vi "Sand Fall Till the Void.vi"(3 "Possible Movements":cdb[](array[numeric]), 4 "Sand Source Coordinates":cdb, 5 "Rock Grid":set{cdb}(c389)) -> (0 "Bounds":T1, 1 "Sand Fall steps":T2(array[cluster]), 2 "Sand Grid":set{cdb}(c389))   [LabVIEW 2020, in "AoC 2022.lvlib"]
uses:
  AoC 2022.lvlib
panel:
  out "size":i32
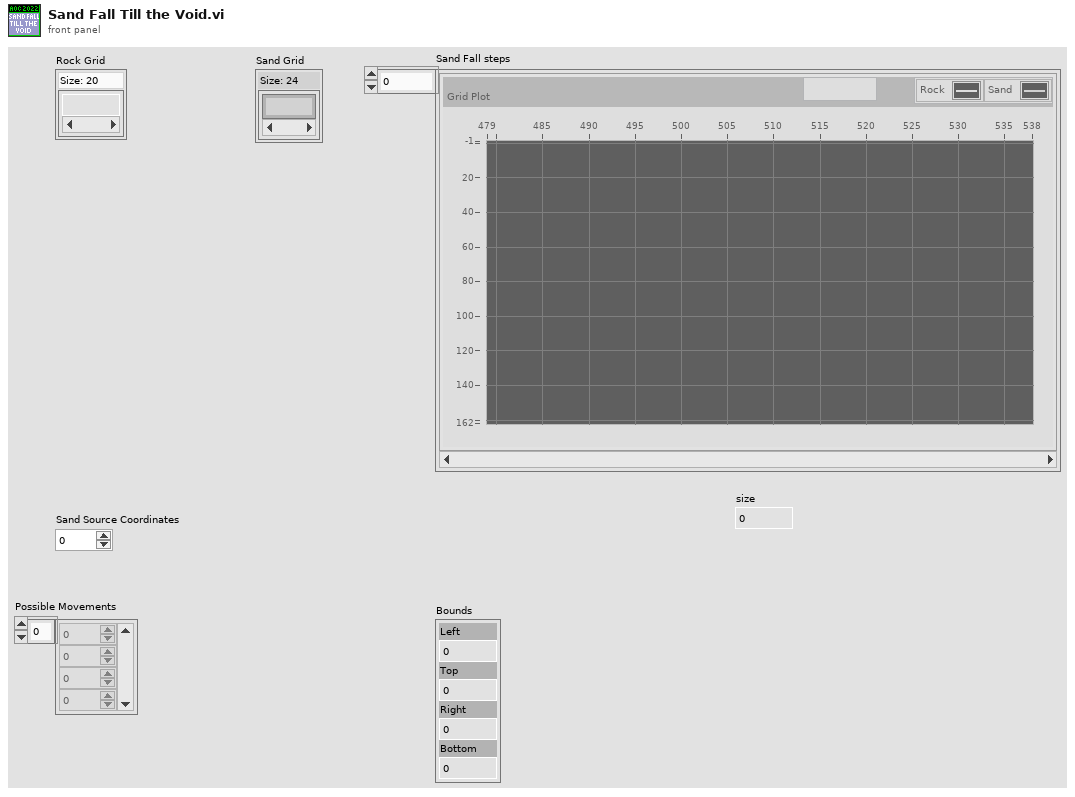
[diagram p1: front panel]
types:
  T1 = cluster{"Left":i16, "Top":i16, "Right":i16, "Bottom":i16}
  T2 = cluster{"Grid Plot":cluster{cluster{i32, i32}[]}[]}[]
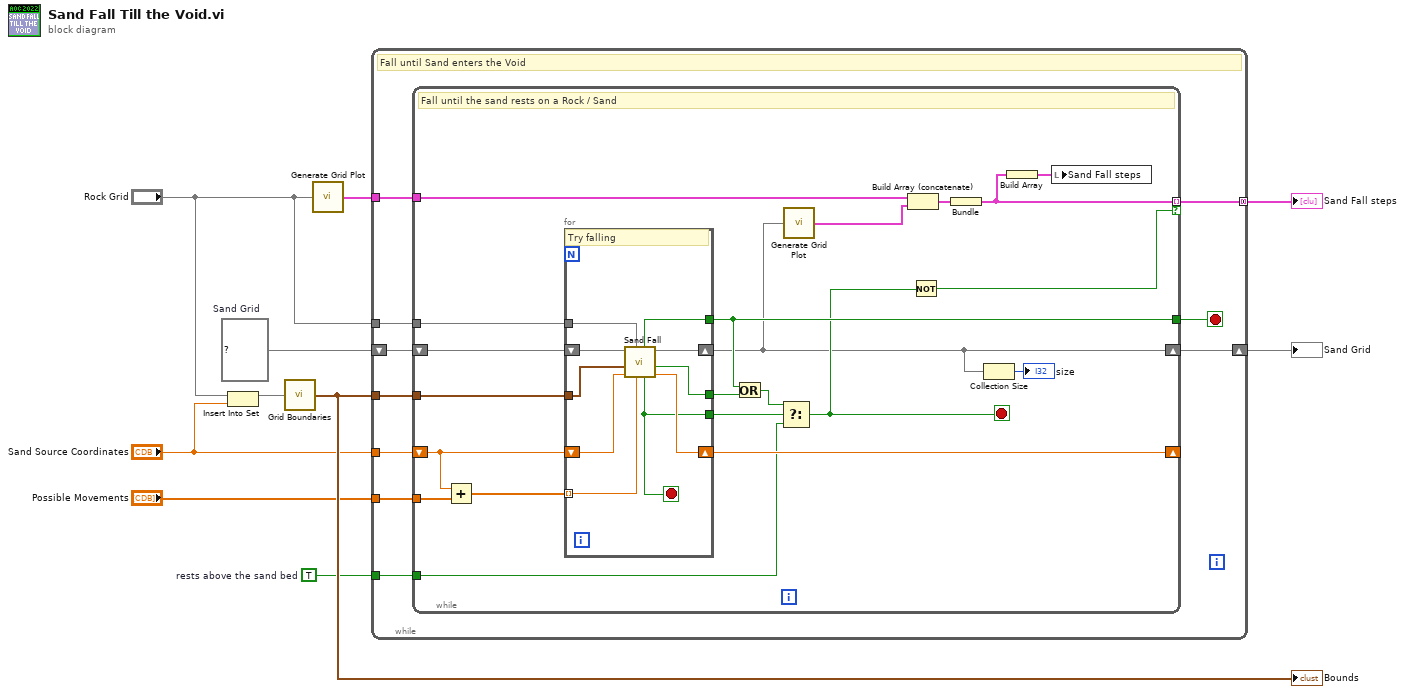
[diagram p0: block diagram]
diagram:
  w1 = TRUE  # rests above the sand bed
  w2 = set{cdb} {}  # Sand Grid
  n1 = Insert Into Set(10:"Sand Source Coordinates", 11:"Rock Grid") -> (3:w4:set{cdb})  [unwired: 1 out]
  n2 = call "Grid Boundaries.vi"("Grid"=w4) -> ("Bounds"=w9:T1)
  "Bounds" <- w9
  n3 = call "Generate Grid Plot.vi"("Grid"="Rock Grid") -> ("Grid Plot"=w7:cluster{cluster{i32, i32}[]}[])
  n4 = while {
    tunnel: "Rock Grid" -> [w17]
    shift-right: [w12] -> w8
    shift-left: w2 -> [w18]
    tunnel: "Sand Source Coordinates" -> [w20]
    tunnel: w9 -> [w19]
    tunnel: "Possible Movements" -> [w16]
    tunnel: w7 -> [w14]
    tunnel: [w13] -> w10 mode=concatenating
    tunnel: w1 -> [w11]
    stop <- w15 stop-if-true
    # "Fall until Sand enters the Void"
    n5 = while {
      tunnel: w19 -> [w38]
      shift-right: [w22] -> w12
      shift-left: w18 -> [w40]
      shift-right: [w41] -> _
      shift-left: w20 -> [w39]
      tunnel: w17 -> [w31]
      tunnel: w16 -> [w37]
      tunnel: [w34] -> w15
      tunnel: w14 -> [w30]
      tunnel: [w24] -> w13 mode=indexing if=w27
      tunnel: w11 -> [w26]
      stop <- w28 stop-if-true
      # "Fall until the sand rests on a Rock / Sand"
      n6 = Add(x=w39, y=w37) -> (x+y=w36:cdb[])
      n7 = for {
        tunnel: w31 -> [w49]
        tunnel: w38 -> [w47]
        shift-right: [w48] -> w41
        shift-left: w39 -> [w46]
        shift-right: [w51] -> w22
        shift-left: w40 -> [w50]
        tunnel: w36 -> [w45] mode=indexing
        tunnel: [w44] -> w35
        tunnel: [w43] -> w34
        tunnel: [w42] -> w33
        stop <- w42 stop-if-true
        # "Try falling"
        n8 = call "Sand Fall.vi"("Next Location"=w45, "Rock Grid"=w49, "Current Location in"=w46, "Bounds"=w47, "Sand Grid in"=w50) -> ("Current Location out"=w48:cdb, "Sand Reached Resting Position ?"=w44:bool, "Sand Grid out"=w51:set{cdb}, "Arrived at Decision ?"=w42:bool, "Falling into Void ?"=w43:bool)  [unwired: 2 in]
      }
      n9 = Or(x=w34, y=w35) -> (x .or. y?=w32:bool)
      n10 = Select(t=w32, s=w33, f=w26) -> (s? t:f=w28:bool)
      n11 = call "Generate Grid Plot.vi"("Grid"=w22) -> ("Grid Plot"=w29:cluster{cluster{i32, i32}[]}[])
      n12 = Build Array (concatenate)(w30, w29) -> (w25:cluster{cluster{i32, i32}[]}[])
      n13 = Not(x=w28) -> (.not. x?=w27:bool)
      n14 = Bundle(w25) -> (w24:cluster{cluster{cluster[]}[]})  [unwired: 1 in]
      n15 = Collection Size(1:w22) -> (0:→"size":i32)
      n16 = Build Array(w24) -> (w23:cluster{cluster{cluster[]}[]}[])
      n17 = local write "Sand Fall steps"(w23) -> ()
    }
  }
  "Sand Fall steps" <- w10
  "Sand Grid" <- w8
